vi "FullAlign.vi"(0 "Joystick 0":dbl, 5 "Joystick 1":dbl, 7 "Distance":dbl, 9 "Angle":dbl, 11 "Button":bool=TRUE) -> (4 "Right Motor":dbl, 6 "Left Motor":dbl, 15 "output cluster":T1)   [LabVIEW 2016]
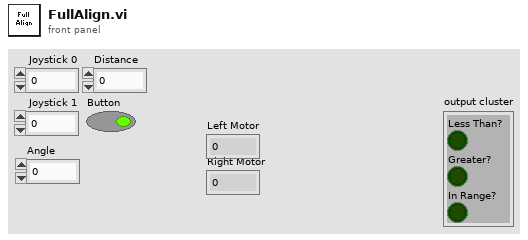
[diagram p1: front panel]
types:
  T1 = cluster{"Less Than? ":bool, "Greater?":bool, "In Range?":bool}
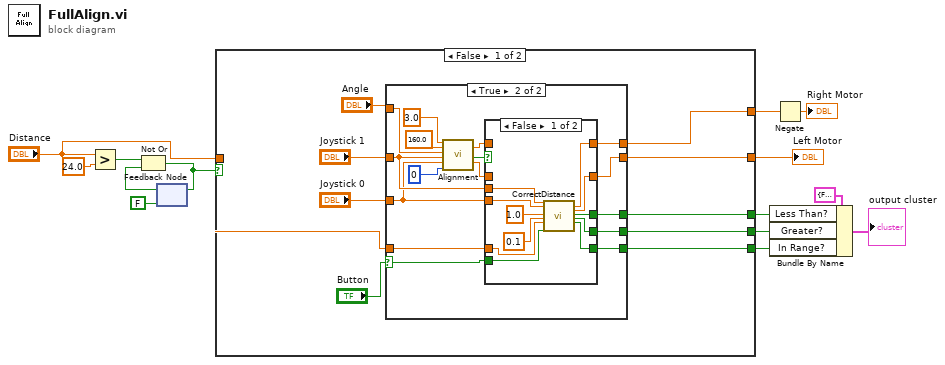
[diagram p0: block diagram]
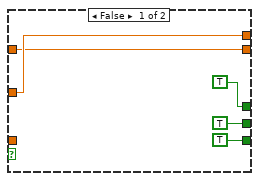
[diagram p2: hidden frame]
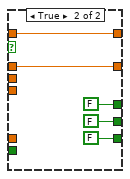
[diagram p3: hidden frame]
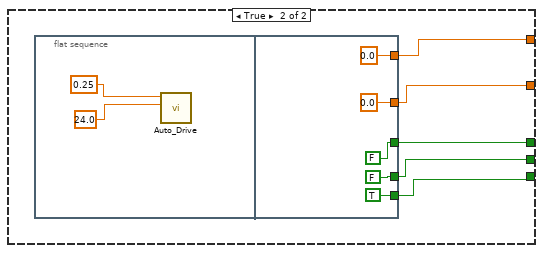
[diagram p4: hidden frame]
diagram:
  n1 = Greater?(x="Distance", y=24.0) -> (0:w8:bool)
  n2 = feedback #1(FALSE) -> (w9:bool)
  n3 = Not Or(1:w9, 2:w8) -> (0:w7:bool)
  n4 = feedback-in #1(w7) -> ()
  n5 = case shown="False" w7 {
    tunnel: "Distance" -> [w20 _]
    tunnel: [w19 w63] -> w5
    tunnel: [w18 w62] -> w4
    tunnel: [w17 w66] -> w3
    tunnel: [w16 w65] -> w2
    tunnel: [w15 w64] -> w1
    frame False {
      n6 = case shown="True" "Button" {
        selector: "Button" -> [_ w35]
        tunnel: "Joystick 1" -> [w28 w40]
        tunnel: "Joystick 0" -> [w29 w39]
        tunnel: [w28 w45] -> w18
        tunnel: [w29 w44] -> w19
        tunnel: "Angle" -> [_ w42]
        tunnel: [TRUE w34] -> w16
        tunnel: [TRUE w33] -> w17
        tunnel: [TRUE w32] -> w15
        tunnel: w20 -> [_ w31]
        frame False {
        }
        frame True {
          n7 = call "Alignment.vi"("Range"=3.0, "Target"=160.0, "Gyroscope Angle"=w42, "RightMotorSpeed"=w40, "LeftMotorSpeed"=w39, "POV"=0) -> ("Right Motor"=w38:dbl, "LeftAndRight?"=w36:bool, "Left Motor"=w37:dbl)  [unwired: 11 in]
          n8 = case shown="False" w36 {
            tunnel: w40 -> [w52 _]
            tunnel: w39 -> [w53 _]
            tunnel: [w51 w60] -> w45
            tunnel: [w50 w61] -> w44
            tunnel: w35 -> [w54 _]
            tunnel: w38 -> [_ w61]
            tunnel: w37 -> [_ w60]
            tunnel: [w49 FALSE] -> w34
            tunnel: [w48 FALSE] -> w33
            tunnel: [w47 FALSE] -> w32
            tunnel: w31 -> [w46 _]
            frame False {
              n9 = call "CorrectDistance.vi"("JoyStick 1"=w52, "JoyStick 2"=w53, "CenterPoint"=1.0, "Range"=0.1, "Distance"=w46, "Button"=w54) -> ("Right Motor"=w50:dbl, "Left Motor"=w51:dbl, "Less than"=w48:bool, "Greater"=w49:bool, "In Range?"=w47:bool)  [unwired: 16 in, 1 out]
            }
            frame True {
            }
          }
        }
      }
    }
    frame True {
      n10 = flat-sequence {
        tunnel: [FALSE] -> w66
        tunnel: [FALSE] -> w65
        tunnel: [TRUE] -> w64
        tunnel: [0.0] -> w63
        tunnel: [0.0] -> w62
        frame #0 {
          n11 = call "Auto_Drive.vi"("distance"=24.0, "Drive Effort"=0.25) -> ()  [unwired: 10 in]
        }
        frame #1 {
        }
      }
    }
  }
  "Left Motor" <- w4
  n12 = Bundle By Name(cluster=T1 {"Less Than? "=FALSE, "Greater?"=FALSE, "In Range?"=FALSE} ("input cluster"), "Less Than?"=w3, "Greater?"=w2, "In Range?"=w1) -> (→"output cluster":T1)
  n13 = Negate(x=w5) -> (-x=→"Right Motor":dbl)
